vi "ResMirror_Delay.vi"(1 "Amplitude (V)":dbl=1.0, 2 "FPGA AQ Clock Speed (MHz)":dbl=200.0, 3 "Mirror Frequency (kHz)":dbl=16.208) -> (0 "Acquisition Delay (Ticks)":u16)   [LabVIEW 2014]
panel:
  out "Acquisition Delay (us)":dbl
  out "Turn Around Delay (us)":dbl
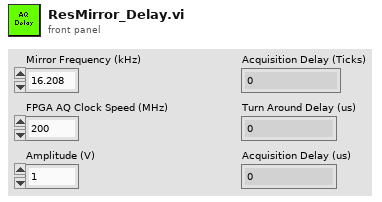
[diagram p1: front panel]
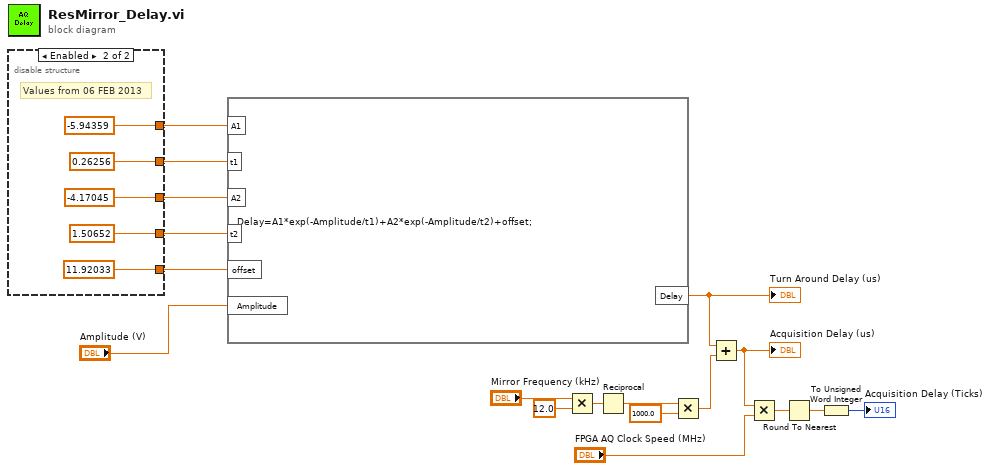
[diagram p0: block diagram]
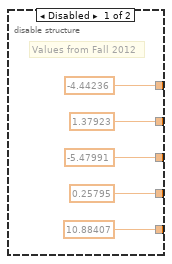
[diagram p2: hidden frame]
diagram:
  n1 = disable-structure shown="Enabled" {
    disable-tunnel: [-4.44236 ("input variable") -5.94359 ("input variable")] -> w18
    disable-tunnel: [1.37923 ("input variable") 0.26256 ("input variable")] -> w17
    disable-tunnel: [-5.47991 ("input variable") -4.17045 ("input variable")] -> w16
    disable-tunnel: [0.25795 ("input variable") 1.50652 ("input variable")] -> w15
    disable-tunnel: [10.88407 ("input variable") 11.92033 ("input variable")] -> w14
    frame Disabled {
      # "Values from Fall 2012"
    }
    frame Enabled {
      # "Values from 06 FEB 2013"
    }
  }
  n2 = formula code="Delay=A1*exp(-Amplitude/t1)+A2*exp(-Amplitude/t2)+offset;"("A1"=w18, "t1"=w17, "A2"=w16, "t2"=w15, "offset"=w14, "Amplitude"="Amplitude (V)") -> ("Delay"=w7:dbl)
  "Turn Around Delay (us)" <- w7
  n3 = Multiply(x="Mirror Frequency (kHz)", y=12.0) -> (x*y=w11:dbl)
  n4 = Reciprocal(x=w11) -> (1/x=w8:dbl)
  n5 = Multiply(x=w8, y=1000.0) -> (x*y=w6:dbl)
  n6 = Add(x=w7, y=w6) -> (x+y=w5:dbl)
  "Acquisition Delay (us)" <- w5
  n7 = Multiply(x=w5, y="FPGA AQ Clock Speed (MHz)") -> (x*y=w4:dbl)
  n8 = Round To Nearest(number=w4) -> (nearest integer value=w2:dbl)
  n9 = To Unsigned Word Integer(number=w2) -> (unsigned 16bit integer=→"Acquisition Delay (Ticks)":u16)
